vi "Write JSON Config.vi"(6 "Pretty Print?":bool, 8 "error in (no error)":errorcluster, 11 "Const_WFM in":refnum<class "Const_WFM.lvclass">) -> (0 "error out":errorcluster, 2 "JSON":string, 3 "Const_WFM out":refnum<class "Const_WFM.lvclass">)   [LabVIEW 2021, in "Const_WFM.lvclass"]
uses:
  Const_WFM.lvclass
  C:/Program Files (x86)/National Instruments/LabVIEW 2021/vi.lib/TSA/Abstract Data Classes/Abs_Types/Type/Abs_Type.lvclass
  Const_WFM.lvclass/Const_WFM.ctl
  410041d9-c61b-43ca-875f-6d5b7e88acad.vi
  <vilib>/Utility/LVClass/Get LV Class Name.vi
  <vilib>/JDP Science/JSONtext/Variant to JSON Text.vi
  <vilib>/JDP Science/JSONtext/Set Multiple Object Items.vi
  <vilib>/JDP Science/JSONtext/LVClass Serializer/JSONtext LVClass Serializer.lvclass
  Abs_Types/Waveform/Abs_Waveform.lvclass
  Abs_Types/Type/Abs_Type.lvclass
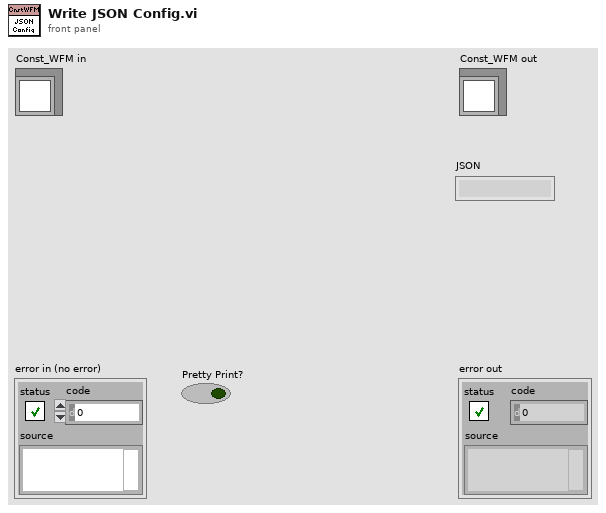
[diagram p1: front panel]
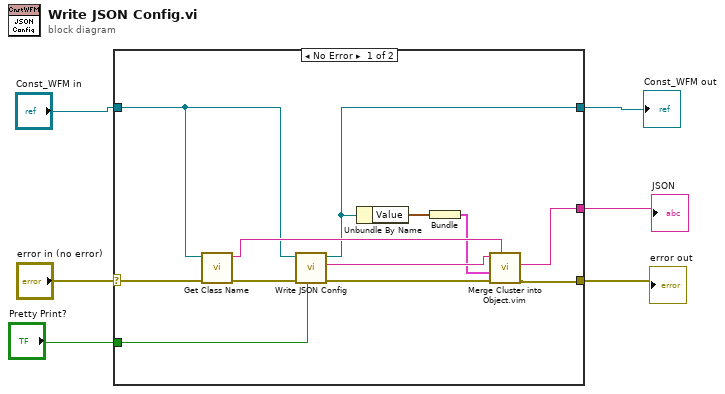
[diagram p0: block diagram]
diagram:
  n1 = case shown="No Error" "error in (no error)" {
    selector: "error in (no error)" -> [w17 w20]
    tunnel: [w14 w20] -> w6
    tunnel: [w9 _] -> w1
    tunnel: [w11 w19] -> w3
    tunnel: "Const_WFM in" -> [w13 w19]
    tunnel: "Pretty Print?" -> [w12 _]
    frame No Error {
      n2 = call "Get Class Name.vi"("error in (no error)"=w17, "Abs_Type in"=w13) -> ("error out"=w18:errorcluster, "class name"=w15:string)  [unwired: 8 in]
      n3 = call-parent "Write JSON Config.vi"("Pretty Print?"=w12, "error in (no error)"=w18, "Abs_Type in"=w13) -> ("error out"=w16:errorcluster, "JSON"=w10:string, "Abs_Type out"=w11:refnum<class "Const_WFM.lvclass">)  [unwired: 6 in]
      n4 = Unbundle By Name(w11) -> ("Value"=w7:waveform(dbl))
      n5 = Bundle("Value"=w7) -> (w8:cluster{"Value":waveform(dbl)})  [unwired: 1 in]
      n6 = call "Merge Cluster into Object.vim"("$Path or Item Name"=w15, "error in (no error)"=w16, "Any Cluster"=w8, "JSON"=w10) -> ("error out"=w14:errorcluster, "<JSON>"=w9:string)  [unwired: 5 in]
    }
    frame Error {
    }
  }
  "error out" <- w6
  "Const_WFM out" <- w3
  "JSON" <- w1
